vi "Check Range.vi"(9 "listbox":i32, 11 "all obj":refnum<class "_ISerializable.lvclass">[](array[class])) -> (3 "_ISerializable out":refnum<class "_ISerializable.lvclass">)   [LabVIEW 2018]
uses:
  _Serializable Base Object/_ISerializable.lvclass
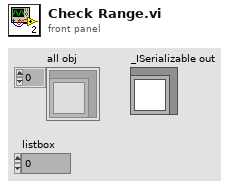
[diagram p1: front panel]
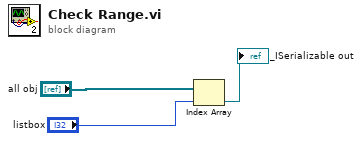
[diagram p0: block diagram]
diagram:
  n1 = Index Array(array="all obj", index="listbox") -> (element=→"_ISerializable out":refnum<class "_ISerializable.lvclass">)
